vi "reactors_notifier.vi"() -> (0 "error out":errorcluster, 3 "Notifier out":refnum<notifier>)   [LabVIEW 2013]
uses:
  main_machine/type_defs/reactors.ctl
  main_machine/type_defs/reactor.ctl
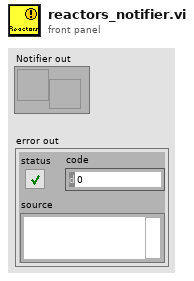
[diagram p1: front panel]
types:
  T1 = typedef "reactors.ctl" = cluster{i32, "TIME STAMPS":dbl[], "LAST MEASUREMENT":T2[][], "SUMMARY STAT":dbl[]}[]
  T2 = typedef "reactor.ctl" = dbl
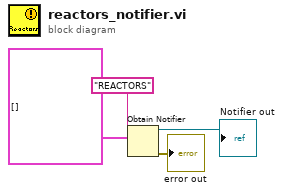
[diagram p0: block diagram]
diagram:
  n1 = Obtain Notifier(name (unnamed)="REACTORS", notification data type=T1 [] ("REACTORS")) -> (notifier out=→"Notifier out":refnum<notifier>, error out=→"error out":errorcluster)  [unwired: 2 in, 1 out]
